vi "FTW-Test-Reflection-CompositeTypes.vi"() -> (0 "Test Result":errorcluster)   [LabVIEW 2015]
uses:
  src/reflection/FTW-Reflection-Types.ctl
  src/reflection/FTW-Reflection-Array.vi
  src/error/FTW-ERR-ThrowInfo.vi
  src/error/FTW-ERR-ThrowError.vi
  src/error/FTW-ERR-CallChain.vi
  src/error/FTW-ERR-NoErrorConstant.vi
  src/string/FTW-STR-ReplaceWhitespace.vi
  src/string/FTW-STR-Array-Delimit.vi
  src/error/FTW-ERR-Clear.vi
  src/regex/FTW-Regex-ReplaceAll.vi
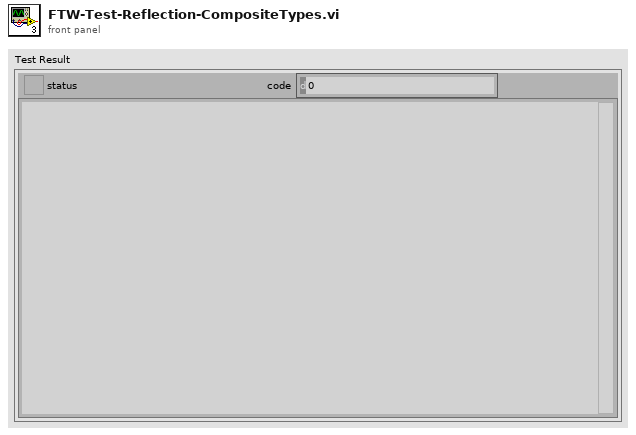
[diagram p1: front panel]
types:
  T1 = cluster{"Timestamp":timestamp, "LVVariant":variant}
  T2 = cluster{"VIReference":refnum<vi>, "ApplicationInstance":refnum<vi>, "VIServerReference (Generic Class)":refnum<vi>}
  T3 = cluster{"ConnectionIrDA":refnum<k19>, "ConnectionTCP":refnum<k5>, "ConnectionUDP":refnum<k16>, "ConnectionBluetooth":refnum<k31>, "ConnectionDataSocket":refnum<k13>}
  T4 = cluster{"Notifier":refnum<notifier>, "Queue":refnum<queue>, "EventPublisher":refnum<user-event>, "DataValueReference":refnum<data-value>, "Occurrence":refnum<k4>, "EventCallback":refnum<k27>, "EventRegistration":refnum<event-registration>}
  T5 = cluster{"String":string, "Picture":picture, "Path":path, "ConnectionVISA":refnum<visa-resource-name>, "GenericClassTag (Shared Variable Reference)":refnum<k21>, "GenericClassTag (Network Stream Endpoint)":refnum<k21>}
  T6 = cluster{"FileByteStream":refnum<file>, "GenericClass (DOM XML)":refnum<k20>, "TDMStream":refnum<k34>, "OverloadedDatalogRef (Mouse Input Device)":refnum<k1>, "GenericClass (storage refnum)":refnum<k20>, "dotNET":refnum<k24>, "ActiveX":refnum<k7>, "Menu":refnum<k9>}
  T7 = cluster{"WaveformU8":waveform(u8), "WaveformU16":waveform(u16), "WaveformU32":waveform(u32), "WaveformU64":waveform(u64), "WaveformI8":waveform(i8), "WaveformI16":waveform(i16), "WaveformI32":waveform(i32), "WaveformI64":waveform(i64), "WaveformSGL":waveform(sgl), "WaveformDBL":waveform(dbl), "WaveformEXT":waveform(ext), "WaveformCSG":waveform(csg), "WaveformCDB":waveform(cdb), "WaveformCXT":waveform(cxt), "WaveformDigital":digitalwaveform, "DynamicData":dynamicdata, "DigitalData":digitaldata}
  T8 = cluster{"Cluster":cluster{"I32":i32}, "LVObject":refnum<class>}
  T9 = cluster{"Array":i32[], "ByteArray":u8[], "Array 2":cluster{"I32":i32}[]}
  T10 = typedef "FTW-Reflection-Types.ctl" = enum16{"Unknown", "Void", "Array", "Cluster", "LVObject", "Boolean", "I8", "I16", "I32", "I64", "U8", "U16", "U32", "U64", "SGL", "DBL", "EXT", "CSG", "CDB", "CXT", "FXP", "EnumU8", "EnumU16", "EnumU32", "EnumU64", "SGLwithUnit", "DBLwithUnit", "EXTwithUnit", "CSGwithUnit", "CDBwithUnit", "CXTwithUnit", "String", "Path", "Picture", "Tag", "LVVariant", "Timestamp", "WaveformI8", "WaveformI16", "WaveformI32", "WaveformI64", "WaveformU8", "WaveformU16", "WaveformU32", "WaveformU64", "WaveformSGL", "WaveformDBL", "WaveformEXT", "WaveformCSG", "WaveformCDB", "WaveformCXT", "WaveformDigital", "WaveformUnknownType", "DigitalData", "DynamicData", "ExternalData", "FileByteStream", "TDMStream", "dotNET", "ActiveX", "VIServerReference", "VIReference", "ApplicationInstance", "Menu", "ConnectionDataSocket", "ConnectionVISA", "ConnectionBluetooth", "ConnectionIrDA", "ConnectionTCP", "ConnectionUDP", "ConnectionHTTPClient", "ConnectionFTP", "Occurrence", "Notifier", "Queue", "Rendezvous", "Semaphore", "RTFIFO", "EventPublisher", "EventRegistration", "EventCallback", "DataValueReference", "GenericClass", "GenericClassTag", "GenericClassDeepCopy", "GenericClassFlattened", "GenericClassTagFlattened", "GenericReferenceType", "WindowsRegistry", "OverloadedDatalogRef", "ReferenceUnknownType", "ByteArray", "ConPaneInterface"}
  T11 = cluster{"EnumU8":enum8{"U8"}, "EnumU16":enum16{"U16"}, "EnumU32":enum32{"U32"}, "EnumU32 (Enum U64 doesn't yet exist!)":enum32{"U64"}, "EnumU16 (FTW-Reflection-Types.ctl)":T10}
  T12 = cluster{"SGLwithUnit":sgl[unit], "DBLwithUnit":dbl[unit], "EXTwithUnit":ext[unit], "CSGwithUnit":csg[unit], "CDBwithUnit":cdb[unit], "CXTwithUnit":cxt[unit]}
  T13 = cluster{"SGL":sgl, "DBL":dbl, "EXT":ext, "CSG":csg, "CDB":cdb, "CXT":cxt, "FXP":fxp<+/-,64,1024>}
  T14 = cluster{"U8":u8, "U16":u16, "U32":u32, "U64":u64, "I8":i8, "I16":i16, "I32":i32, "I64":i64}
  T15 = cluster{"Element Name":string, "Element Type":T10, "Element Value":variant}[]
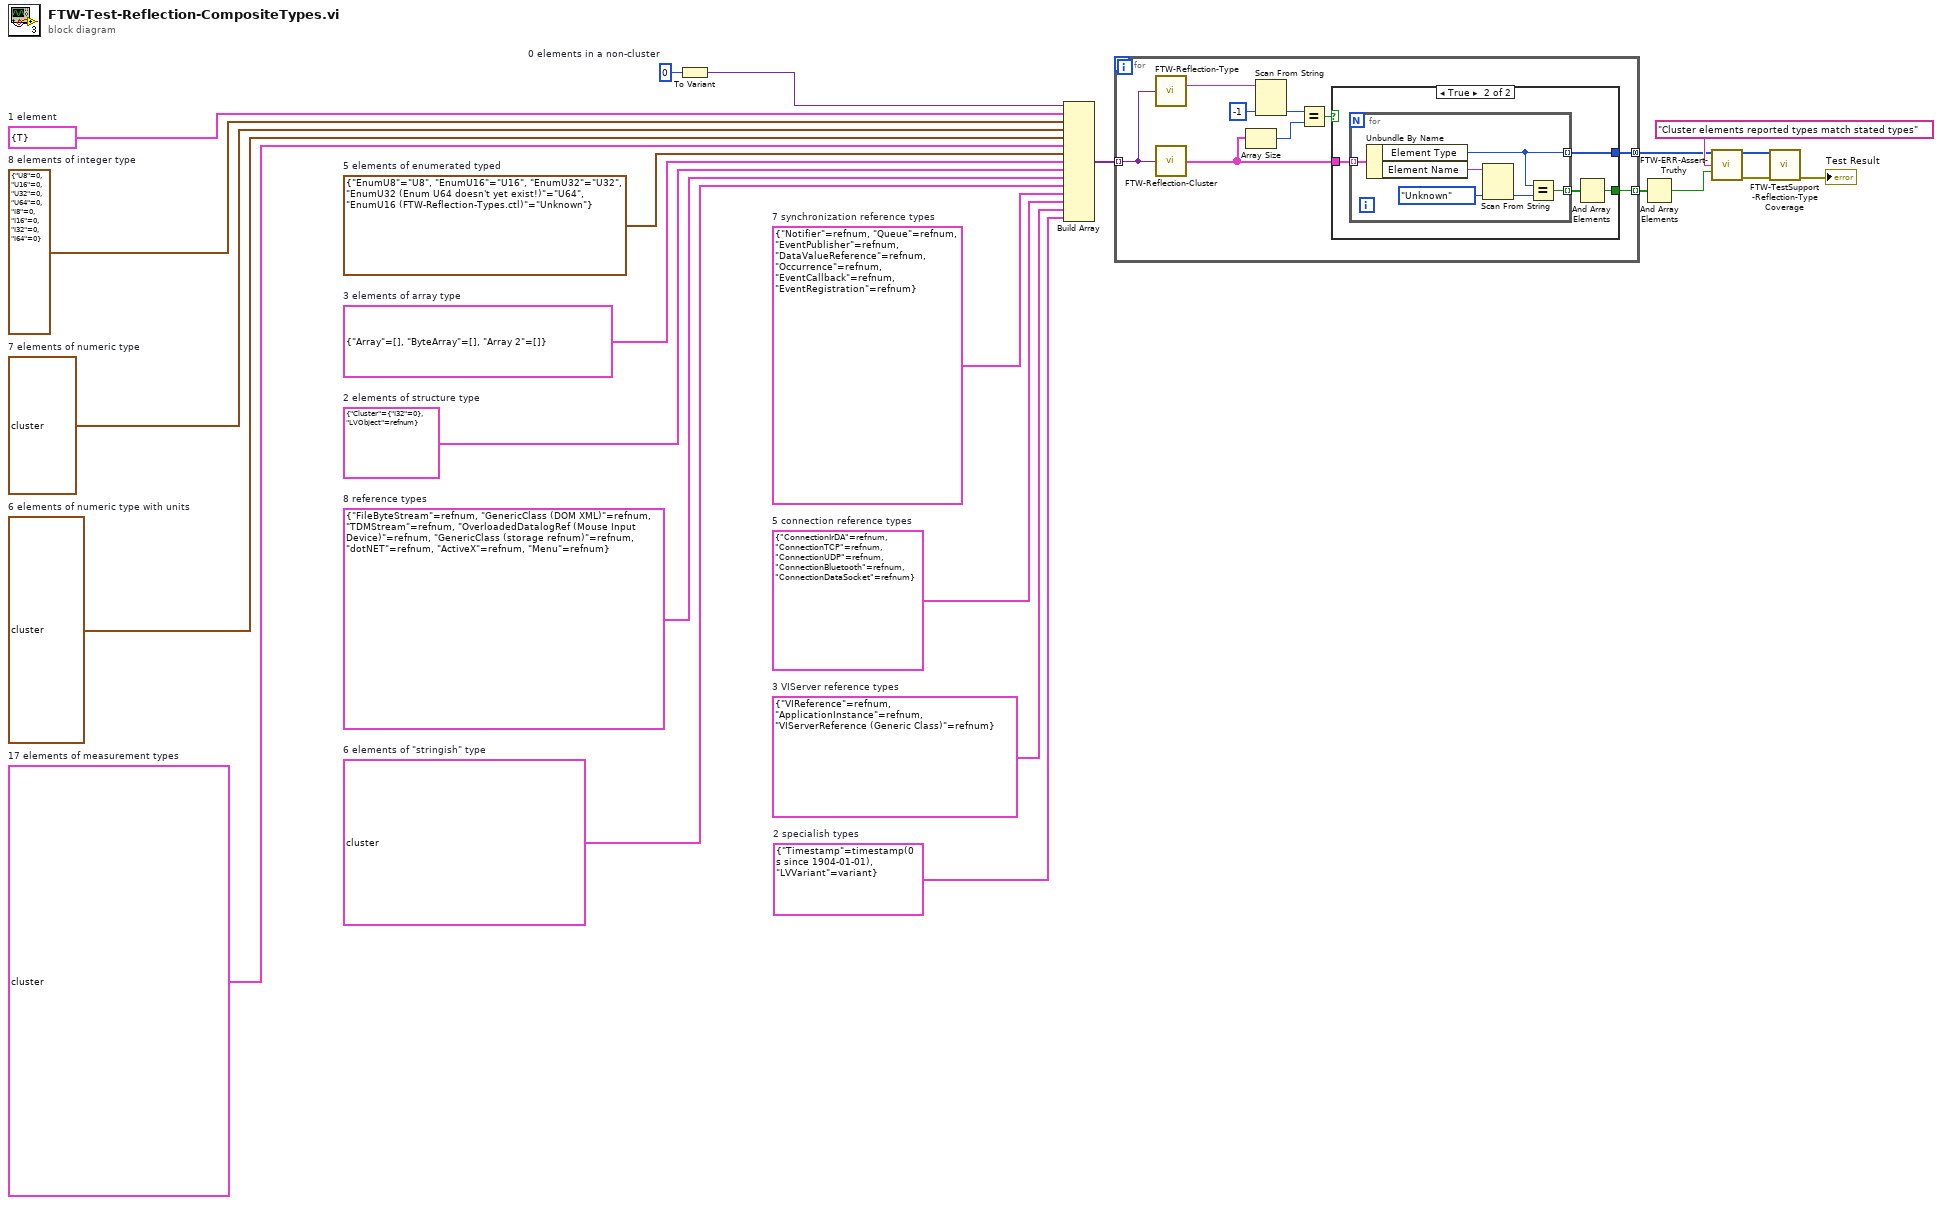
[diagram p0: block diagram]
diagram:
  w4 = T1 {"Timestamp"=timestamp(0 s since 1904-01-01), "LVVariant"=variant}  # 2 specialish types
  w6 = T2 {"VIReference"=refnum, "ApplicationInstance"=refnum, "VIServerReference (Generic Class)"=refnum}  # 3 VIServer reference types
  w7 = T3 {"ConnectionIrDA"=refnum, "ConnectionTCP"=refnum, "ConnectionUDP"=refnum, "ConnectionBluetooth"=refnum, "ConnectionDataSocket"=refnum}  # 5 connection reference types
  w8 = T4 {"Notifier"=refnum, "Queue"=refnum, "EventPublisher"=refnum, "DataValueReference"=refnum, "Occurrence"=refnum, "EventCallback"=refnum, "EventRegistration"=refnum}  # 7 synchronization reference types
  w11 = 0  # 0 elements in a non-cluster
  w5 = T5 {"String"="", "Picture"=bytes[0], "Path"=path "", "ConnectionVISA"="", "GenericClassTag (Shared Variable Reference)"="ni.var.psp://localhost/System", "GenericClassTag (Network Stream Endpoint)"="localhost"}  # 6 elements of "stringish" type
  w13 = T6 {"FileByteStream"=refnum, "GenericClass (DOM XML)"=refnum, "TDMStream"=refnum, "OverloadedDatalogRef (Mouse Input Device)"=refnum, "GenericClass (storage refnum)"=refnum, "dotNET"=refnum, "ActiveX"=refnum, "Menu"=refnum}  # 8 reference types
  w9 = T7 {"WaveformU8"={"t0"=timestamp(0 s since 1904-01-01), "dt"=1.0, "Y"=[]}, "WaveformU16"={"t0"=timestamp(0 s since 1904-01-01), "dt"=1.0, "Y"=[]}, "WaveformU32"={"t0"=timestamp(0 s since 1904-01-01), "dt"=1.0, "Y"=[]}, "WaveformU64"={"t0"=timestamp(0 s since 1904-01-01), "dt"=1.0, "Y"=[]}, "WaveformI8"={"t0"=timestamp(0 s since 1904-01-01), "dt"=1.0, "Y"=[]}, "WaveformI16"={"t0"=timestamp(0 s since 1904-01-01), "dt"=1.0, "Y"=[]}, "WaveformI32"={"t0"=timestamp(0 s since 1904-01-01), "dt"=1.0, "Y"=[]}, "WaveformI64"={"t0"=timestamp(0 s since 1904-01-01), "dt"=1.0, "Y"=[]}, "WaveformSGL"={"t0"=timestamp(0 s since 1904-01-01), "dt"=1.0, "Y"=[]}, "WaveformDBL"={"t0"=timestamp(0 s since 1904-01-01), "dt"=1.0, "Y"=[]}, "WaveformEXT"={"t0"=timestamp(0 s since 1904-01-01), "dt"=1.0, "Y"=[]}, "WaveformCSG"={"t0"=timestamp(0 s since 1904-01-01), "dt"=1.0, "Y"=[]}, "WaveformCDB"={"t0"=timestamp(0 s since 1904-01-01), "dt"=1.0, "Y"=[]}, "WaveformCXT"={"t0"=timestamp(0 s since 1904-01-01), "dt"=1.0, "Y"=[]}, "WaveformDigital"={"t0"=timestamp(0 s since 1904-01-01), "dt"=0.0, "Y"={"transitions"=[], "data"=[]}}, "DynamicData"=[], "DigitalData"={"transitions"=[], "data"=[]}}  # 17 elements of measurement types
  w14 = T8 {"Cluster"={"I32"=0}, "LVObject"=refnum}  # 2 elements of structure type
  w15 = T9 {"Array"=[], "ByteArray"=[], "Array 2"=[]}  # 3 elements of array type
  w16 = T11 {"EnumU8"=enum."U8", "EnumU16"=enum."U16", "EnumU32"=enum."U32", "EnumU32 (Enum U64 doesn't yet exist!)"=enum."U64", "EnumU16 (FTW-Reflection-Types.ctl)"=enum."Unknown"}  # 5 elements of enumerated typed
  w19 = T12 {"SGLwithUnit"=0.0, "DBLwithUnit"=0.0, "EXTwithUnit"=0.0, "CSGwithUnit"=0.0+0.0i, "CDBwithUnit"=0.0+0.0i, "CXTwithUnit"=0.0+0.0i}  # 6 elements of numeric type with units
  w20 = T13 {"SGL"=0.0, "DBL"=0.0, "EXT"=0.0, "CSG"=0.0+0.0i, "CDB"=0.0+0.0i, "CXT"=0.0+0.0i, "FXP"=0.0}  # 7 elements of numeric type
  w21 = T14 {"U8"=0, "U16"=0, "U32"=0, "U64"=0, "I8"=0, "I16"=0, "I32"=0, "I64"=0}  # 8 elements of integer type
  w10 = cluster{"Boolean":bool} {"Boolean"=TRUE}  # 1 element
  n1 = To Variant(anything=w11) -> (Variant=w12:variant)
  n2 = Build Array(w12, w10, w21, w20, w19, w9, w16, w15, w14, w13, w5, w8, w7, w6, w4) -> (w23:variant[])
  n3 = for {
    tunnel: w23 -> [w32] mode=indexing
    tunnel: [w25] -> w22 mode=indexing
    tunnel: [w24] -> w1 mode=concatenating
    n4 = call "FTW-Reflection-Type.vi"("Anything"=w32) -> ("Data Name"=w31:string)  [unwired: 12 in, 2 out]
    n5 = call "FTW-Reflection-Cluster.vi"("Cluster"=w32) -> ("Cluster Elements"=w29:T15)  [unwired: 14 in]
    n6 = Array Size(array=w29) -> (size(s)=w27:i32)
    n7 = Scan From String(input string=w31, default 1=-1 ("default value 1")) -> (output 1=w28:i32)  [unwired: 3 in, 3 out]
    n8 = Equal?(x=w28, y=w27) -> (x = y?=w26:bool)
    n9 = case shown="True" w26 {
      tunnel: w29 -> [_ w36]
      tunnel: [_ w34] -> w25
      tunnel: [_ w33] -> w24
      frame False {
      }
      frame True {
        n10 = for {
          tunnel: w36 -> [w42] mode=indexing
          tunnel: [w39] -> w35 mode=indexing
          tunnel: [w37] -> w33 mode=indexing
          n11 = Unbundle By Name(w42) -> ("Element Type"=w37:T10, "Element Name"=w38:string)
          n12 = Scan From String(input string=w38, default 1=FTW-Reflection-Types."Unknown" ("Element Type")) -> (output 1=w40:T10)  [unwired: 3 in, 3 out]
          n13 = Equal?(x=w37, y=w40) -> (x = y?=w39:bool)
        }
        n14 = And Array Elements(Boolean array=w35) -> (logical AND=w34:bool)
      }
    }
  }
  n15 = And Array Elements(Boolean array=w22) -> (logical AND=w3:bool)
  n16 = call "FTW-ERR-Assert-Truthy.vi"("Assertion"="Cluster elements reported types match stated types", "Assertion holds true?"=w3) -> ("error out"=w18:errorcluster)  [unwired: 13 in]
  n17 = call "FTW-TestSupport-Reflection-TypeCoverage.vi"("Types Tested"=w1, "error in"=w18) -> ("error out"=→"Test Result":errorcluster)  [unwired: 13 in]
